vi "ScopeReadout_writeFile.vi"() -> ()   [LabVIEW 2016]
doc: "Example: Configured Acquisition Auto TRIG\n\nRecommended Input Signal: 100 kHz, 4 Vpp, sine wave\n\nDevices Supported: NI 5102, NI 5911, NI 5112, NI 5620 \n(NI 5620 requires configuring 50 ohm input impedance and a 2 V vertical range)\n\nDescription:\n\nThis example is the same as the configured acquisition example included with the shipping examples, except this VI will use an immediate trigger if a timeout error is returned because no trigger is present. If a timeout occurs the code aborts and resets the session, while setting the trigger source to immediate. This example allows you use any of the available trigger sources, rather than just edge trigger as in the AutoSetup VI."
uses:
  <instrlib>/niScope/Acquire/Fetch/niScope Multi Fetch.vi
panel:
  out "Histogram":dynamicdata(graph)
  in  "resource name":refnum<k15>="PXI1Slot8"
  in  "Operator":string="Hsin-Yeh"
  in  "Target Total Events":i32=10000
  in  "file path":path=path "C:/Users/NTU/Desktop/Chih-Ping/NaI0827/1-haveNumber/Co60/Co60_5.tdms"
  out "Waveform from Digitizer vs. Sample Number":dbl[][](graph)=[[-0.007034295140918245, -0.005815471424873819, -0.004596647708829393, -0.0033778239927849674, -0.0033778239927849674, -0.004596647708829393, -0.007034295140918245, -0.0033778239927849674, -0.005815471424873819, -0.0033778239927849674, -0.0021590002767405414, -0.005815471424873819, -0.005815471424873819, -0.004596647708829393, -0.005815471424873819, -0.004596647708829393, -0.007034295140918245, -0.0021590002767405414, -0.005815471424873819, -0.005815471424873819, -0.0033778239927849674, -0.004596647708829393, -0.004596647708829393, -0.004596647708829393, -0.0033778239927849674, -0.0021590002767405414, -0.007034295140918245, -0.004596647708829393, -0.0033778239927849674, -0.004596647708829393, -0.0021590002767405414, -0.007034295140918245, -0.004596647708829393, -0.005815471424873819, -0.0033778239927849674, -0.0033778239927849674, -0.004596647708829393, -0.004596647708829393, -0.005815471424873819, -0.004596647708829393, -0.008253118856962671, -0.004596647708829393, -0.004596647708829393, -0.004596647708829393, -0.004596647708829393, -0.007034295140918245, -0.007034295140918245, -0.005815471424873819, -0.007034295140918245, -0.004596647708829393, -0.005815471424873819, -0.004596647708829393, -0.004596647708829393, -0.0021590002767405414, -0.007034295140918245, 0.0002786471553483105, -0.005815471424873819, -0.005815471424873819, -0.0033778239927849674, -0.005815471424873819, -0.004596647708829393, -0.004596647708829393, -0.005815471424873819, -0.005815471424873819, -0.005815471424873819, -0.005815471424873819, -0.0033778239927849674, -0.007034295140918245, -0.004596647708829393, -0.004596647708829393, -0.004596647708829393, -0.0033778239927849674, -0.005815471424873819, -0.0033778239927849674, -0.004596647708829393, -0.005815471424873819, -0.005815471424873819, -0.0021590002767405414, -0.004596647708829393, -0.004596647708829393, -0.004596647708829393, -0.0033778239927849674, -0.009471942573007097, -0.004596647708829393, -0.007034295140918245, -0.004596647708829393, -0.007034295140918245, -0.0033778239927849674, -0.0033778239927849674, -0.004596647708829393, -0.005815471424873819, -0.0021590002767405414, -0.005815471424873819, -0.005815471424873819, -0.004596647708829393, -0.004596647708829393, -0.007034295140918245, -0.0033778239927849674, -0.005815471424873819, -0.008253118856962671, -0.007034295140918245, -0.004596647708829393, -0.0033778239927849674, -0.004596647708829393, -0.008253118856962671, -0.0033778239927849674, -0.007034295140918245, -0.0033778239927849674, -0.0033778239927849674, -0.004596647708829393, -0.007034295140918245, -0.004596647708829393, -0.0033778239927849674, -0.007034295140918245, -0.004596647708829393, -0.004596647708829393, -0.007034295140918245, -0.004596647708829393, -0.005815471424873819, -0.004596647708829393, -0.007034295140918245, -0.004596647708829393, -0.004596647708829393, -0.0033778239927849674, -0.005815471424873819, -0.007034295140918245, -0.005815471424873819, -0.005815471424873819, -0.004596647708829393, -0.005815471424873819, -0.004596647708829393, -0.0033778239927849674, -0.0033778239927849674, -0.005815471424873819, -0.005815471424873819, -0.004596647708829393, -0.004596647708829393, -0.005815471424873819, -0.004596647708829393, -0.005815471424873819, -0.005815471424873819, -0.0021590002767405414, -0.0033778239927849674, -0.004596647708829393, -0.007034295140918245, -0.005815471424873819, -0.005815471424873819, -0.004596647708829393, -0.007034295140918245, -0.005815471424873819, -0.0033778239927849674, -0.0009401765606961154, -0.004596647708829393, -0.004596647708829393, -0.0033778239927849674, -0.0021590002767405414, -0.005815471424873819, -0.004596647708829393, -0.005815471424873819, 0.008810413167659292, 0.06000100924152518, 0.07584571755010272, 0.08559630727845813, 0.08803395471054698, 0.09169042585868026, 0.08803395471054698, 0.0892527784265914, 0.08803395471054698, 0.09169042585868026, 0.09290924957472468, 0.0892527784265914, 0.08803395471054698, 0.09047160214263583, 0.0892527784265914, 0.09169042585868026, 0.08681513099450255, 0.0892527784265914, 0.08803395471054698, 0.08559630727845813, 0.08681513099450255, 0.0892527784265914, 0.08803395471054698, 0.08315865984636928, 0.08559630727845813, 0.08559630727845813, 0.08559630727845813, 0.08315865984636928, 0.08559630727845813, 0.0843774835624137, 0.08315865984636928, 0.08193983613032485, 0.08315865984636928, 0.0843774835624137, 0.079502188698236, 0.08315865984636928, 0.079502188698236, 0.0843774835624137, 0.0843774835624137, 0.079502188698236, 0.07828336498219157, 0.08072101241428042, 0.079502188698236, 0.07828336498219157, 0.079502188698236, 0.07706454126614715, 0.07706454126614715, 0.079502188698236, 0.079502188698236, 0.07828336498219157, 0.0746268938340583, 0.07828336498219157, 0.07584571755010272, 0.07218924640196944, 0.079502188698236, 0.07340807011801387, 0.07584571755010272, 0.0746268938340583, 0.07340807011801387, 0.07218924640196944, 0.07340807011801387, 0.07218924640196944, 0.07340807011801387, 0.07097042268592502, 0.07097042268592502, 0.0746268938340583, 0.07218924640196944, 0.07097042268592502, 0.07340807011801387, 0.06975159896988059, 0.06853277525383616, 0.07340807011801387, 0.06731395153779174, 0.07097042268592502, 0.06975159896988059, 0.07097042268592502, 0.06853277525383616, 0.06853277525383616, 0.06731395153779174, 0.06731395153779174, 0.06609512782174731, 0.06609512782174731, 0.06609512782174731, 0.06975159896988059, 0.06487630410570289, 0.06487630410570289, 0.06731395153779174, 0.06609512782174731, 0.06487630410570289, 0.062438656673614035, 0.06365748038965846, 0.06731395153779174, 0.06731395153779174, 0.062438656673614035, 0.06000100924152518, 0.06121983295756961, 0.06121983295756961, 0.06365748038965846, 0.06365748038965846, 0.062438656673614035, 0.06000100924152518, 0.062438656673614035, 0.06121983295756961, 0.05878218552548076, 0.05878218552548076, 0.06121983295756961, 0.05878218552548076, 0.06121983295756961, 0.06000100924152518, 0.06000100924152518, 0.05756336180943633, 0.05878218552548076, 0.05878218552548076, 0.056344538093391905, 0.056344538093391905, 0.05756336180943633, 0.06000100924152518, 0.05756336180943633, 0.05878218552548076, 0.06000100924152518, 0.056344538093391905, 0.056344538093391905, 0.05512571437734748, 0.05512571437734748, 0.05512571437734748, 0.05512571437734748, 0.05512571437734748, 0.05268806694525863, 0.05390689066130305, 0.05268806694525863, 0.05512571437734748, 0.0514692432292142, 0.05390689066130305, 0.0514692432292142, 0.05268806694525863, 0.05268806694525863, 0.05268806694525863, 0.0514692432292142, 0.050250419513169775, 0.04903159579712535, 0.04903159579712535, 0.04903159579712535, 0.050250419513169775, 0.05268806694525863, 0.050250419513169775, 0.050250419513169775, 0.050250419513169775, 0.0514692432292142, 0.044156300932947645, 0.0514692432292142, 0.0465939483650365, 0.0514692432292142, 0.0465939483650365, 0.04903159579712535, 0.050250419513169775, 0.044156300932947645, 0.04903159579712535, 0.04781277208108092, 0.04781277208108092, 0.04903159579712535, 0.0465939483650365, 0.04171865350085879, 0.0465939483650365, 0.04537512464899207, 0.0465939483650365, 0.044156300932947645, 0.04781277208108092, 0.04537512464899207, 0.044156300932947645, 0.044156300932947645, 0.04781277208108092, 0.04171865350085879, 0.04171865350085879, 0.04293747721690322, 0.04293747721690322, 0.04171865350085879, 0.044156300932947645, 0.04293747721690322, 0.04171865350085879, 0.038062182352725515, 0.04537512464899207, 0.04293747721690322, 0.04049982978481437, 0.04293747721690322, 0.03928100606876994, 0.04293747721690322, 0.04049982978481437, 0.04171865350085879, 0.03928100606876994, 0.04049982978481437, 0.04049982978481437, 0.04049982978481437, 0.04171865350085879, 0.04049982978481437, 0.03928100606876994, 0.03928100606876994, 0.03928100606876994, 0.04171865350085879, 0.04049982978481437, 0.038062182352725515, 0.03684335863668109, 0.03684335863668109, 0.03928100606876994, 0.038062182352725515, 0.035624534920636663, 0.038062182352725515, 0.03928100606876994, 0.038062182352725515, 0.03684335863668109, 0.03318688748854781, 0.03928100606876994, 0.03684335863668109, 0.03318688748854781, 0.035624534920636663, 0.035624534920636663, 0.03684335863668109, 0.03440571120459224, 0.03684335863668109, 0.035624534920636663, 0.03440571120459224, 0.03440571120459224, 0.03684335863668109, 0.03318688748854781, 0.035624534920636663, 0.03318688748854781, 0.038062182352725515, 0.035624534920636663, 0.035624534920636663, 0.03440571120459224, 0.03318688748854781, 0.03440571120459224, 0.03440571120459224, 0.03318688748854781, 0.03318688748854781, 0.03318688748854781, 0.03318688748854781, 0.03318688748854781, 0.03074924005645896, 0.03074924005645896, 0.029530416340414534, 0.029530416340414534, 0.03318688748854781, 0.031968063772503386, 0.028311592624370108, 0.031968063772503386, 0.029530416340414534, 0.03074924005645896, 0.027092768908325682, 0.03074924005645896, 0.03074924005645896, 0.031968063772503386, 0.031968063772503386, 0.027092768908325682, 0.029530416340414534, 0.03074924005645896, 0.02465512147623683, 0.028311592624370108, 0.029530416340414534, 0.029530416340414534, 0.029530416340414534, 0.03074924005645896, 0.027092768908325682, 0.028311592624370108, 0.027092768908325682, 0.029530416340414534, 0.027092768908325682, 0.02465512147623683, 0.031968063772503386, 0.027092768908325682, 0.027092768908325682, 0.027092768908325682, 0.02465512147623683, 0.028311592624370108, 0.02465512147623683, 0.025873945192281256, 0.025873945192281256, 0.023436297760192404, 0.027092768908325682, 0.023436297760192404, 0.025873945192281256, 0.025873945192281256, 0.02465512147623683, 0.028311592624370108, 0.027092768908325682, 0.027092768908325682, 0.023436297760192404, 0.022217474044147978, 0.025873945192281256, 0.02465512147623683, 0.023436297760192404, 0.027092768908325682, 0.023436297760192404, 0.023436297760192404, 0.022217474044147978, 0.027092768908325682, 0.02465512147623683, 0.02465512147623683, 0.02465512147623683, 0.023436297760192404, 0.02465512147623683, 0.02465512147623683, 0.02465512147623683, 0.022217474044147978, 0.02465512147623683, 0.02465512147623683, 0.02465512147623683, 0.02465512147623683, 0.022217474044147978, 0.022217474044147978, 0.020998650328103552, 0.017342179179970274, 0.020998650328103552, 0.019779826612059126, 0.020998650328103552, 0.0185610028960147, 0.022217474044147978, 0.020998650328103552, 0.023436297760192404, 0.019779826612059126, 0.019779826612059126, 0.022217474044147978, 0.017342179179970274, 0.0185610028960147, 0.0185610028960147, 0.019779826612059126, 0.014904531747881422, 0.019779826612059126, 0.02465512147623683, 0.019779826612059126, 0.019779826612059126, 0.020998650328103552, 0.019779826612059126, 0.016123355463925848, 0.019779826612059126, 0.020998650328103552, 0.017342179179970274, 0.0185610028960147, 0.0185610028960147, 0.017342179179970274, 0.0185610028960147, 0.020998650328103552, 0.0185610028960147, 0.019779826612059126, 0.017342179179970274, 0.014904531747881422, 0.016123355463925848, 0.017342179179970274, 0.0185610028960147, 0.016123355463925848, 0.017342179179970274, 0.017342179179970274, 0.017342179179970274, 0.0185610028960147, 0.019779826612059126, 0.014904531747881422, 0.019779826612059126, 0.013685708031836996, 0.016123355463925848, 0.017342179179970274, 0.014904531747881422, 0.017342179179970274, 0.016123355463925848, 0.017342179179970274, 0.014904531747881422, 0.014904531747881422, 0.013685708031836996, 0.017342179179970274, 0.016123355463925848, 0.013685708031836996, 0.017342179179970274, 0.0185610028960147, 0.014904531747881422, 0.016123355463925848, 0.013685708031836996, 0.017342179179970274, 0.01246688431579257, 0.014904531747881422, 0.014904531747881422, 0.014904531747881422, 0.014904531747881422, 0.014904531747881422, 0.013685708031836996, 0.013685708031836996, 0.016123355463925848, 0.01246688431579257, 0.013685708031836996, 0.013685708031836996, 0.013685708031836996, 0.013685708031836996, 0.014904531747881422, 0.014904531747881422, 0.01246688431579257, 0.01246688431579257, 0.013685708031836996, 0.014904531747881422, 0.013685708031836996, 0.013685708031836996, 0.013685708031836996, 0.01246688431579257, 0.017342179179970274, 0.016123355463925848, 0.013685708031836996, 0.016123355463925848, 0.01246688431579257, 0.013685708031836996, 0.014904531747881422, 0.01246688431579257, 0.010029236883703718, 0.013685708031836996, 0.010029236883703718, 0.010029236883703718, 0.014904531747881422, 0.013685708031836996, 0.014904531747881422, 0.011248060599748144, 0.008810413167659292, 0.011248060599748144, 0.01246688431579257, 0.013685708031836996, 0.008810413167659292, 0.013685708031836996, 0.01246688431579257, 0.01246688431579257, 0.01246688431579257, 0.01246688431579257, 0.008810413167659292, 0.013685708031836996, 0.013685708031836996, 0.010029236883703718, 0.008810413167659292, 0.011248060599748144, 0.01246688431579257, 0.01246688431579257, 0.008810413167659292, 0.01246688431579257, 0.010029236883703718, 0.013685708031836996, 0.00637276573557044, 0.007591589451614866, 0.010029236883703718, 0.010029236883703718, 0.010029236883703718, 0.008810413167659292, 0.01246688431579257, 0.011248060599748144, 0.010029236883703718, 0.008810413167659292, 0.008810413167659292, 0.011248060599748144, 0.007591589451614866, 0.010029236883703718, 0.008810413167659292, 0.00637276573557044, 0.008810413167659292, 0.01246688431579257, 0.008810413167659292, 0.01246688431579257, 0.011248060599748144, 0.008810413167659292, 0.008810413167659292, 0.007591589451614866, 0.008810413167659292, 0.00637276573557044, 0.010029236883703718, 0.010029236883703718, 0.005153942019526014, 0.00637276573557044, 0.007591589451614866, 0.007591589451614866, 0.008810413167659292, 0.008810413167659292, 0.010029236883703718, 0.008810413167659292, 0.008810413167659292, 0.007591589451614866, 0.007591589451614866, 0.007591589451614866, 0.00637276573557044, 0.00637276573557044, 0.010029236883703718, 0.00637276573557044, 0.007591589451614866, 0.007591589451614866, 0.010029236883703718, 0.010029236883703718, 0.011248060599748144, 0.008810413167659292, 0.005153942019526014, 0.007591589451614866, 0.00637276573557044, 0.00637276573557044, 0.00637276573557044, 0.005153942019526014, 0.007591589451614866, 0.007591589451614866, 0.007591589451614866, 0.007591589451614866, 0.01246688431579257, 0.00637276573557044, 0.007591589451614866, 0.008810413167659292, 0.005153942019526014, 0.005153942019526014, 0.008810413167659292, 0.00637276573557044, 0.00637276573557044, 0.00637276573557044, 0.005153942019526014, 0.003935118303481588, 0.005153942019526014, 0.007591589451614866, 0.0014974708713927365, 0.005153942019526014, 0.005153942019526014, 0.005153942019526014, 0.007591589451614866, 0.003935118303481588, 0.005153942019526014, 0.003935118303481588, 0.008810413167659292, 0.003935118303481588, 0.003935118303481588, 0.003935118303481588, 0.00637276573557044, 0.005153942019526014, 0.005153942019526014, 0.005153942019526014, 0.005153942019526014, 0.007591589451614866, 0.00637276573557044, 0.00637276573557044, 0.005153942019526014, 0.00637276573557044, 0.00637276573557044, 0.00637276573557044, 0.003935118303481588, 0.003935118303481588, 0.005153942019526014, 0.005153942019526014, 0.005153942019526014, 0.008810413167659292, 0.0027162945874371625, 0.005153942019526014, 0.005153942019526014, 0.0027162945874371625, 0.003935118303481588, 0.005153942019526014, 0.003935118303481588, 0.0014974708713927365, 0.003935118303481588, 0.00637276573557044, 0.005153942019526014, 0.00637276573557044, 0.0027162945874371625, 0.003935118303481588, 0.0027162945874371625, 0.003935118303481588, 0.003935118303481588, 0.0027162945874371625, 0.007591589451614866, 0.005153942019526014, 0.003935118303481588, 0.003935118303481588, 0.005153942019526014, 0.003935118303481588, 0.0027162945874371625, 0.005153942019526014, 0.0027162945874371625, 0.00637276573557044, -0.0009401765606961154, 0.003935118303481588, 0.005153942019526014, 0.005153942019526014, 0.003935118303481588, 0.005153942019526014, 0.0002786471553483105, 0.0002786471553483105, 0.003935118303481588, 0.0014974708713927365, 0.0027162945874371625, 0.0027162945874371625, 0.0014974708713927365, 0.0027162945874371625, 0.0027162945874371625, 0.0014974708713927365, 0.0014974708713927365, 0.003935118303481588, 0.0027162945874371625, 0.0014974708713927365, 0.0027162945874371625, 0.0027162945874371625, 0.0027162945874371625, 0.005153942019526014, 0.0027162945874371625, 0.0014974708713927365, 0.003935118303481588, -0.0021590002767405414, 0.0002786471553483105, 0.005153942019526014, 0.0002786471553483105, 0.0027162945874371625, 0.0027162945874371625, 0.003935118303481588, 0.0027162945874371625, 0.0014974708713927365, -0.0009401765606961154, 0.0002786471553483105, 0.003935118303481588, 0.0002786471553483105, 0.0014974708713927365, 0.005153942019526014, 0.0027162945874371625, 0.0027162945874371625, 0.0027162945874371625, 0.003935118303481588, 0.003935118303481588, 0.0002786471553483105, 0.0027162945874371625, 0.0002786471553483105, 0.0014974708713927365, -0.0021590002767405414, 0.003935118303481588, 0.0027162945874371625, 0.0014974708713927365, 0.0027162945874371625, 0.0002786471553483105, 0.0014974708713927365, 0.0014974708713927365, 0.0002786471553483105, 0.0014974708713927365, 0.0014974708713927365, -0.0009401765606961154, 0.0014974708713927365, 0.0002786471553483105, 0.0014974708713927365, 0.0002786471553483105, 0.0002786471553483105, 0.0014974708713927365, 0.0014974708713927365, 0.0002786471553483105, -0.0009401765606961154]]
  out "Event rate (Hz)":dbl=73.3159330185636
  in  "reference position":dbl=20.0 caption="Ref Position" format="%.1f"
  out "Event Number":dbl=10000.0
  in  "Don't Write Data":bool
  in  "trigger coupling":i32(slide)=1 caption="Trigger Coupling"
  in  "trigger level":dbl=0.03 caption="Trigger Level" format="%.2f"
  in  "trigger holdoff":dbl caption="Trigger Holdoff" format="%^.4e"
  in  "trigger delay":dbl caption="Trigger Delay" format="%^.4e"
  in  "trigger slope":i32(ring) caption="Trigger Slope" items=["Positive", "Negative"]
  in  "trigger source":string(combo)="0" caption="Trigger Source"
  in  "maximum input frequency":dbl=1000000000.0 caption="Max. Input Frequency" format="%.2f"
  in  "input impedance":u32(ring)=2 caption="Input Impedance" items=["1 mega ohm", "75 ohms", "50 ohms"]
  in  "vertical coupling":u32(slide)=1 caption="Vertical\nCcoupling"
  in  "probe attenuation":dbl=1.0 caption="Probe Attenuation" format="%.1f"
  in  "vertical offset":dbl=0.5 caption="Vertical Offset" format="%.4f"
  in  "trigger type":enum16{"Edge"}(ring) caption="Trigger Type"
  out "actual sample rate":dbl=5000000.0 caption="Actual Sample Rate" format="%^.2e"
  out "actual record length":i32=800 caption="Actual Record Length"
  in  "?":bool
  in  "min record length":i32=800 caption="Min. Record Length"
  in  "min sample rate":dbl=5000000.0 caption="Min. Sample Rate" step=1000000.0 format="%^.2e"
  in  "vertical range":dbl=1.0 caption="Vertical Range (V)" format="%.2f"
  in  "channel name":string="0" caption="Channel Name(s)"
  # "Vertical"
  # "Channel"
  # "Trigger"
  # "Specific Parameters - Not all parameters \napply to all trigger types."
  # "Trigger Selection"
  # "Horizontal"
  # "Common Parameters"
  # "NI PXIe 5162 Spec : 1.5 GHz, 5 GS/s, 10-Bit\nhttps://www.ni.com/pdf/manuals/373858j.pdf"
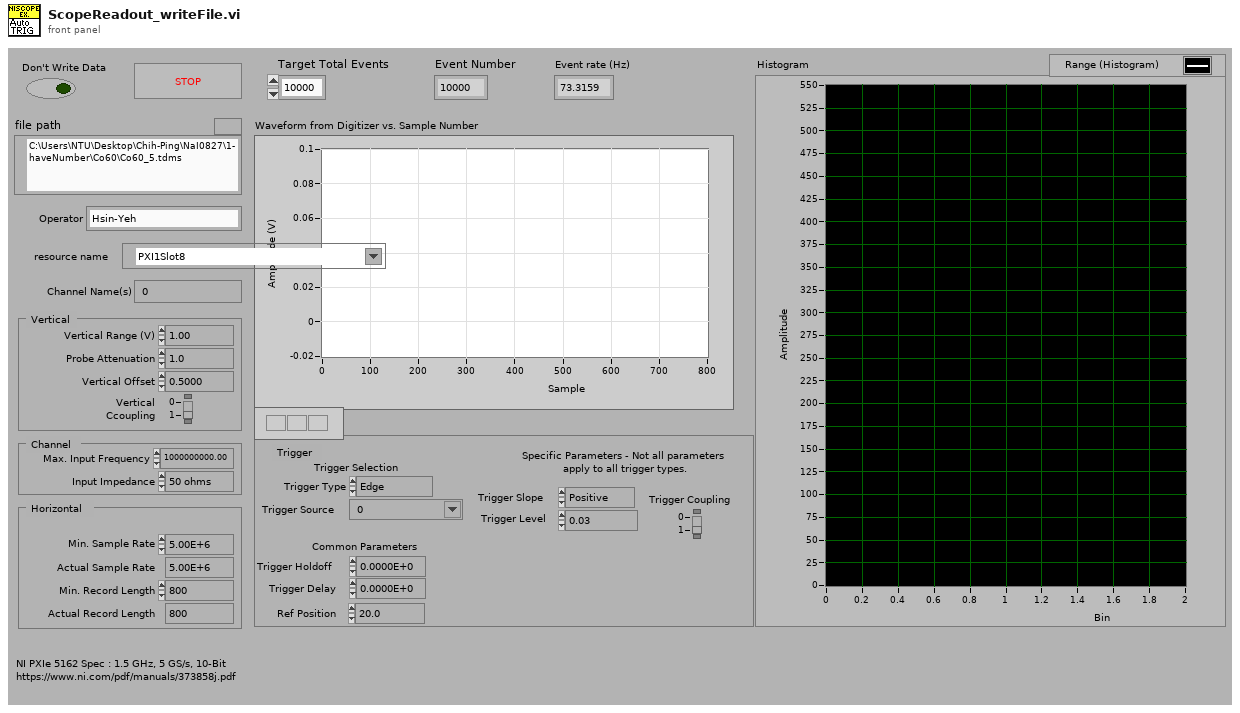
[diagram p1: front panel]
types:
  T1 = enum16{"open", "open or create", "create or replace", "create", "open (read-only)"}
  T2 = enum16{"Edge", "Hysteresis", "Digital", "Window", "Immediate"}
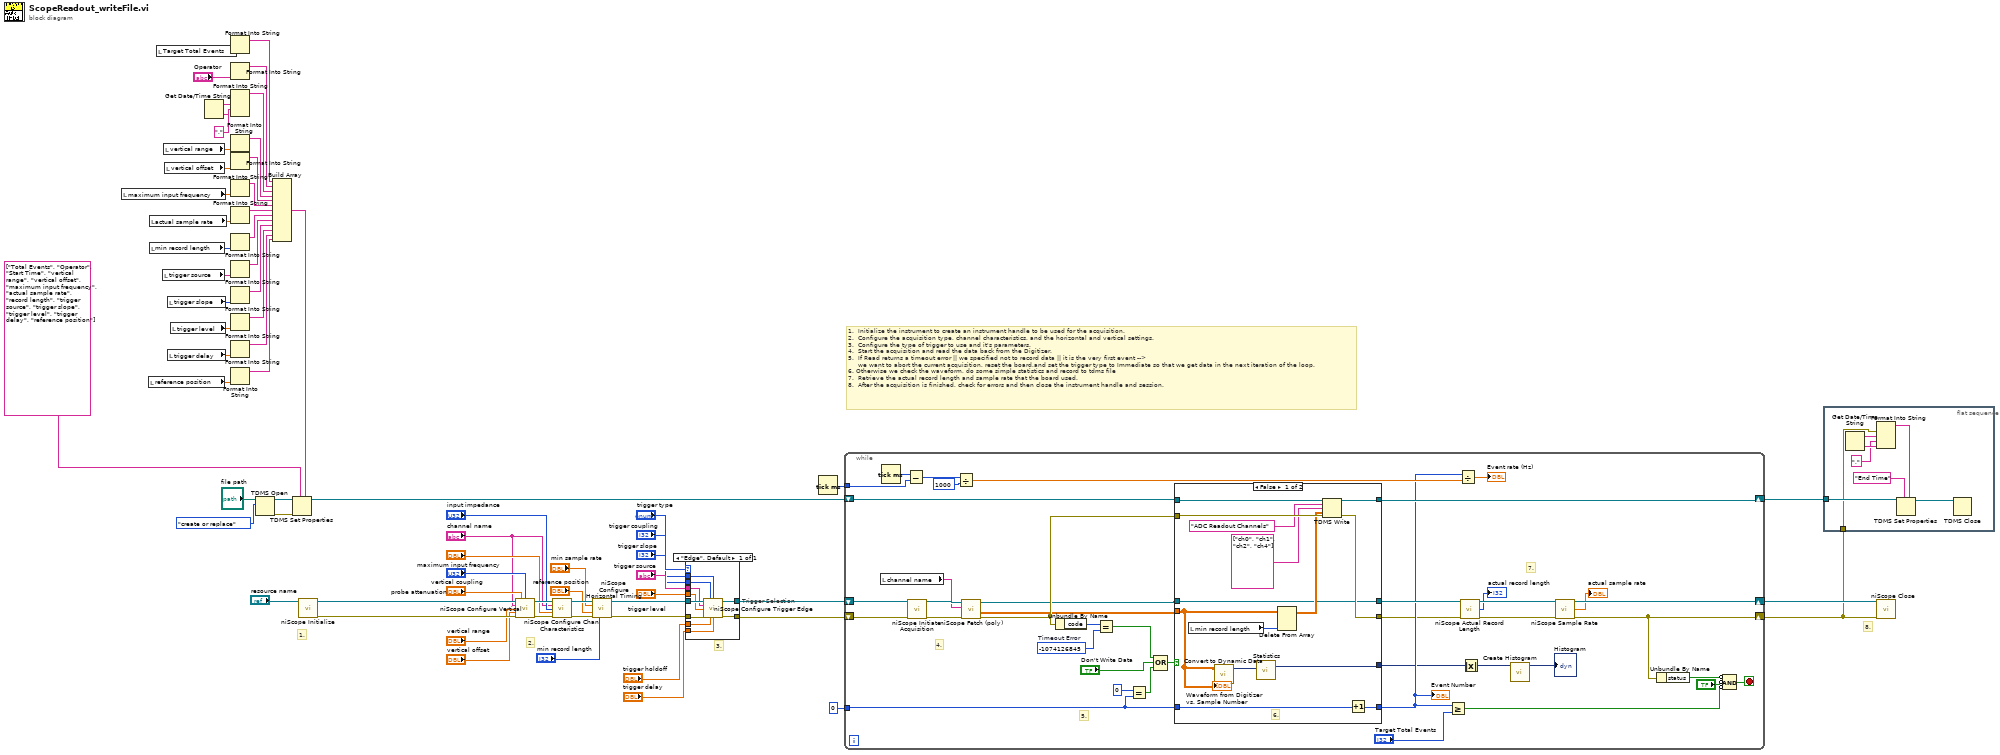
[diagram p0: block diagram]
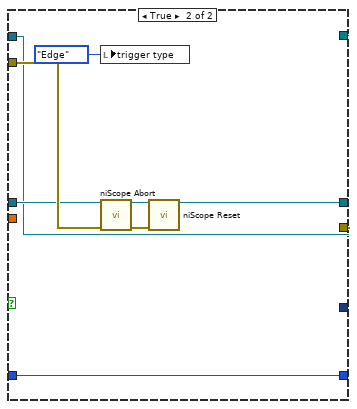
[diagram p2: hidden frame]
diagram:
  # "2."
  # "3."
  # "1.  Initialize the instrument to create an instrument handle to be used for the acquisition.\n2.  Configure the acquisition type, channel characteristics, and the horizontal and vertical settings.\n3.  Configure the type of trigger to use and it's parameters.\n4.  Start the acquisition and read the data back from the Digitizer.\n5.  If Read returns a timeout error || we specified not to record data || it is the very first event -->\n     we want to abort the current acquisition, reset the board,and set the trigger type to Immediate so that we get data in the next iteration of the loop.\n6. Otherwise we check the waveform, do some simple statistics and record to tdms file\n7.  Retrieve the actual record length and sample rate that the board used.\n8.  After the acquisition is finished, check for errors and then close the instrument handle and session."
  # "8."
  # "1."
  n1 = local read "maximum input frequency"() -> (w50:dbl)
  n2 = local read "reference position"() -> (w52:dbl)
  n3 = local read "actual sample rate"() -> (w54:dbl)
  n4 = local read "min record length"() -> (w57:i32)
  n5 = local read "Target Total Events"() -> (w60:i32)
  n6 = local read "trigger source"() -> (w56:string)
  n7 = local read "vertical range"() -> (w55:dbl)
  n8 = local read "vertical offset"() -> (w51:dbl)
  n9 = local read "trigger slope"() -> (w42:i32)
  n10 = local read "trigger delay"() -> (w53:dbl)
  n11 = local read "trigger level"() -> (w58:dbl)
  n12 = Get Date/Time String() -> (date string=w48:string, time string=w46:string)  [unwired: 3 in]
  n13 = Format Into String(w60) -> (resulting string=w59:string)  [unwired: 3 in, 1 out]
  n14 = Format Into String("Operator") -> (resulting string=w45:string)  [unwired: 3 in, 1 out]
  n15 = Format Into String(w48, "," ("input 2"), w46) -> (resulting string=w44:string)  [unwired: 3 in, 1 out]
  n16 = Format Into String(w55) -> (resulting string=w43:string)  [unwired: 3 in, 1 out]
  n17 = Format Into String(w51) -> (resulting string=w40:string)  [unwired: 3 in, 1 out]
  n18 = Format Into String(w50) -> (resulting string=w41:string)  [unwired: 3 in, 1 out]
  n19 = Format Into String(w54) -> (resulting string=w39:string)  [unwired: 3 in, 1 out]
  n20 = Format Into String(w57) -> (resulting string=w38:string)  [unwired: 3 in, 1 out]
  n21 = Format Into String(w56) -> (resulting string=w37:string)  [unwired: 3 in, 1 out]
  n22 = Format Into String(w42) -> (resulting string=w36:string)  [unwired: 3 in, 1 out]
  n23 = Format Into String(w58) -> (resulting string=w35:string)  [unwired: 3 in, 1 out]
  n24 = Format Into String(w53) -> (resulting string=w34:string)  [unwired: 3 in, 1 out]
  n25 = Format Into String(w52) -> (resulting string=w33:string)  [unwired: 3 in, 1 out]
  n26 = TDMS Open(10:T1."create or replace" ("operation (0:open)"), 11:"file path") -> (0:w62:errorcluster, 3:w61:refnum<k34>)  [unwired: 5 in]
  n27 = Build Array(w59, w45, w44, w43, w40, w41, w39, w38, w37, w36, w35, w34, w33) -> (w32:string[])
  n28 = TDMS Set Properties(5:w32, 7:string[] ["Total Events", "Operator", "Start Time", "vertical range", "vertical offset", "maximum input frequency", "actual sample rate", "record length", "trigger source", "trigger slope", "trigger level", "trigger delay", "reference position"] ("property names"), 8:w62, 11:w61) -> (3:w30:refnum<k34>)  [unwired: 2 in, 3 out]
  n29 = call <instrlib>:"niScope Initialize.vi"("resource name"="resource name") -> ("instrument handle"=w68:refnum<k15>, "error out"=w67:errorcluster)  [unwired: 13 in]
  n30 = call <instrlib>:"niScope Configure Vertical.vi"("instrument handle"=w68, "probe attenuation"="probe attenuation", "vertical coupling"="vertical coupling", "channels"="channel name", "vertical range"="vertical range", "vertical offset"="vertical offset", "error in"=w67) -> ("instrument handle out"=w23:refnum<k15>, "error out"=w22:errorcluster)  [unwired: 7 in]
  n31 = call <instrlib>:"niScope Configure Chan Characteristics.vi"("instrument handle"=w23, "channels"="channel name", "input impedance"="input impedance", "maximum input frequency"="maximum input frequency", "error in"=w22) -> ("instrument handle out"=w20:refnum<k15>, "error out"=w21:errorcluster)  [unwired: 9 in]
  n32 = call <instrlib>:"niScope Configure Horizontal Timing.vi"("instrument handle"=w20, "min sample rate"="min sample rate", "reference position"="reference position", "error in"=w21, "min record length"="min record length") -> ("instrument handle out"=w13:refnum<k15>, "error out"=w14:errorcluster)  [unwired: 9 in]
  n33 = case "Trigger Selection" shown="\"Edge\", Default" "trigger type" {
    tunnel: w14 -> [w78]
    tunnel: [w72] -> w1
    tunnel: w13 -> [w77]
    tunnel: [w73] -> w4
    tunnel: "trigger source" -> [w76]
    tunnel: "trigger holdoff" -> [w75]
    tunnel: "trigger delay" -> [w74]
    tunnel: "trigger level" -> [w71]
    tunnel: "trigger slope" -> [w70]
    tunnel: "trigger coupling" -> [w69]
    frame "Edge", Default {
      n34 = call <instrlib>:"niScope Configure Trigger Edge.vi"("instrument handle"=w77, "trigger slope"=w70, "trigger coupling"=w69, "trigger source"=w76, "trigger level"=w71, "error in"=w78, "trigger holdoff"=w75, "trigger delay"=w74) -> ("instrument handle out"=w73:refnum<k15>, "error out"=w72:errorcluster)  [unwired: 6 in]
    }
  }
  n35 = Tick Count (ms)() -> (millisecond timer value=w65:u32)
  n36 = while {
    tunnel: 0 -> [w82]
    tunnel: w65 -> [w119]
    shift-right: [w117] -> w29
    shift-left: w30 -> [w118]
    shift-right: [w116] -> w28
    shift-left: w4 -> [w104]
    shift-right: [w115] -> w27
    shift-left: w1 -> [w92]
    stop <- w84 stop-if-true
    w108 = -1074126845  # Timeout Error
    # "4."
    # "7."
    # "5."
    n37 = local read "channel name"() -> (w93:string)
    n38 = Tick Count (ms)() -> (millisecond timer value=w101:u32)
    n39 = Subtract(x=w101, y=w119) -> (x-y=w100:u32)
    n40 = call <instrlib>:"niScope Initiate Acquisition.vi"("instrument handle"=w104, "error in"=w92) -> ("instrument handle out"=w103:refnum<k15>, "error out"=w91:errorcluster)  [unwired: 12 in]
    n41 = Divide(x=w100, y=u32 1000) -> (x/y=w98:dbl)
    n42 = call-poly <instrlib>:"niScope Fetch (poly).vi"("error in"=w91, "channels"=w93, "instrument handle"=w103) -> ("error out"=w106:errorcluster, "wfm"=w102:dbl[][], "instrument handle out"=w105:refnum<k15>)  [unwired: 5 in, 1 out]
    n43 = Unbundle By Name(w106) -> ("code"=w107:i32)
    n44 = Equal?(x=w107, y=w108) -> (x = y?=w79:bool)
    n45 = Equal?(x=0 ("y"), y=w82) -> (x = y?=w81:bool)
    n46 = Compound Arithmetic op=OR(w79, "Don't Write Data", w81) -> (w95:bool)
    n47 = case shown="False" w95 {
      tunnel: w106 -> [w130 w142]
      tunnel: w105 -> [w123 w141]
      tunnel: [w123 w138] -> w90
      tunnel: [w128 errorcluster {"status"=FALSE, "code"=0, "source"=""} ("error out")] -> w88
      tunnel: w102 -> [w120 _]
      tunnel: [w129 w135] -> w117
      tunnel: w82 -> [w133 w134]
      tunnel: [w132 w134] -> w89
      tunnel: w118 -> [w131 w135]
      tunnel: [w121 _] -> w85
      frame False {
        # "6."
        n48 = local read "min record length"() -> (w124:i32)
        n49 = call "Convert to Dynamic Data"("2D Array"=w120) -> ("Dynamic Data Type"=w122:dynamicdata)  [unwired: 3 in]
        n50 = call "Statistics"("Signals"=w122) -> ("Range"=w121:dynamicdata)  [unwired: 23 in, 3 out]
        n51 = Delete From Array(array=w120, index (col)=w124) -> (array with subset deleted=w125:dbl[][])  [unwired: 2 in, 1 out]
        n52 = TDMS Write(0:w131, 5:"ADC Readout Channels" ("group name (Untitled)"), 7:string[] ["ch0", "ch1", "ch2", "ch4"] ("channel name(s)"), 9:w125, 11:w130) -> (4:w129:refnum<k34>, 15:w128:errorcluster)  [unwired: 1 in, 2 out]
        n53 = Increment(x=w133) -> (x+1=w132:i32)
        "Waveform from Digitizer vs. Sample Number" <- w120
      }
      frame True {
        n54 = local write "trigger type"(T2."Edge" ("trigger type")) -> ()
        n55 = call <instrlib>:"niScope Abort.vi"("instrument handle"=w141, "error in"=w142) -> ("instrument handle out"=w140:refnum<k15>, "error out"=w139:errorcluster)  [unwired: 12 in]
        n56 = call <instrlib>:"niScope Reset.vi"("instrument handle"=w140, "error in"=w139) -> ("instrument handle out"=w138:refnum<k15>)  [unwired: 12 in, 1 out]
      }
    }
    "Event Number" <- w89
    n57 = Greater Or Equal?(x=w89, y="Target Total Events") -> (x >= y?=w94:bool)
    n58 = Divide(x=w89, y=w98) -> (x/y=→"Event rate (Hz)":dbl)
    n59 = call <instrlib>:"niScope Actual Record Length.vi"("instrument handle"=w90, "error in"=w88) -> ("instrument handle out"=w114:refnum<k15>, "actual record length"=→"actual record length":i32, "error out"=w113:errorcluster)  [unwired: 11 in]
    n60 = Absolute Value(x=w85) -> (abs(x)=w86:dynamicdata)
    n61 = call "Create Histogram"("Signal"=w86) -> ("Histogram"=→"Histogram":dynamicdata)  [unwired: 9 in, 1 out]
    n62 = call <instrlib>:"niScope Sample Rate.vi"("instrument handle"=w114, "error in"=w113) -> ("instrument handle out"=w116:refnum<k15>, "actual sample rate"=→"actual sample rate":dbl, "error out"=w115:errorcluster)  [unwired: 11 in]
    n63 = Unbundle By Name(w115) -> ("status"=w109:bool)
    n64 = Compound Arithmetic op=AND(invert w109, invert "?", invert w94) -> (w84:bool)
  }
  n65 = flat-sequence {
    tunnel: w29 -> [w150]
    tunnel: w27 -> [w143]
    frame #0 {
      n66 = Get Date/Time String() -> (date string=w148:string, time string=w147:string)  [unwired: 3 in]
      n67 = Format Into String(error in=w143, w148, "," ("input 2"), w147) -> (resulting string=w145:string)  [unwired: 2 in, 1 out]
      n68 = TDMS Set Properties(5:w145, 7:"End Time" ("input 2"), 11:w150) -> (3:w149:refnum<k34>)  [unwired: 3 in, 3 out]
      n69 = TDMS Close(11:w149) -> ()  [unwired: 1 in, 2 out]
    }
  }
  n70 = call <instrlib>:"niScope Close.vi"("instrument handle"=w28, "error in"=w27) -> ()  [unwired: 13 in, 1 out]
